vi "Keithley 6517 Perform Zero Correction_Cut.vi"(2 "Error In":errorcluster, 3 "VISA resource name":refnum<visa-resource-name>) -> (0 "Error Out":errorcluster, 1 "Measurement":T1 {"Measurement" format="%.6e"})   [LabVIEW 2016]
doc: "This example shows how to perform zero correction.\n\n<B>Note:</B>\nThis Example is compatible with both model 6517 and 6514."
uses:
  <instrlib>/Keithley 6517/Keithley 6517.lvlib
panel:
  in  "Instrument Model":i32(ring)=2 items=["MODEL 6517B", "MODEL 6517A", "MODEL 6514"]
  # "(c) 2016-2017 National Instruments.  ALL RIGHTS RESERVED."
  # "Note: This Example is compatible with model 6517 and 6514."
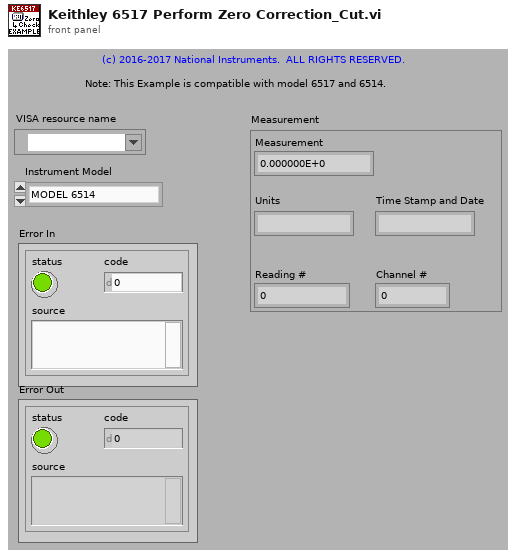
[diagram p1: front panel]
types:
  T1 = cluster{"Measurement":dbl, "Units":string, "Time Stamp and Date":string, "Reading #":dbl, "Channel #":dbl}
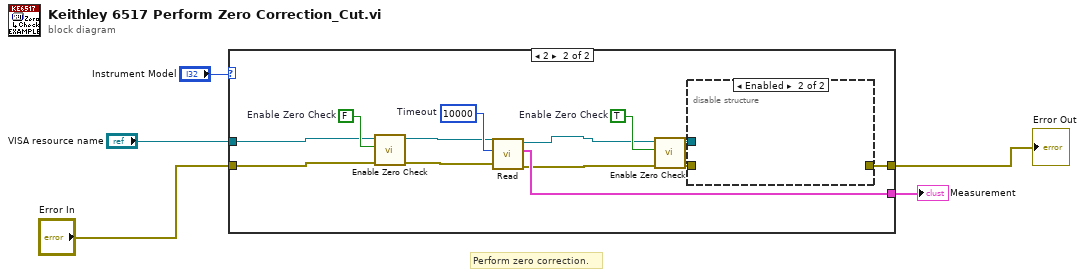
[diagram p0: block diagram]
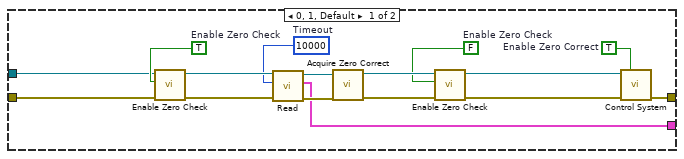
[diagram p2: hidden frame]
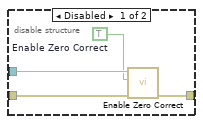
[diagram p3: hidden frame]
diagram:
  # "Perform zero correction."
  n1 = case shown="2" "Instrument Model" {
    tunnel: "VISA resource name" -> [w14 w32]
    tunnel: "Error In" -> [w13 w31]
    tunnel: [w12 w27] -> w1
    tunnel: [w6 w29] -> w5
    frame 0, 1, Default {
      w7 = u32 10000  # Timeout
      w17 = FALSE  # Enable Zero Check
      w20 = TRUE  # Enable Zero Correct
      w21 = TRUE  # Enable Zero Check
      n2 = call <instrlib>:"Enable Zero Check.vi"("error in (no error)"=w13, "Enable Zero Check (T: Enable)"=w21, "VISA resource name"=w14) -> ("error out"=w8:errorcluster, "VISA resource name out"=w9:refnum<visa-resource-name>)  [unwired: 7 in]
      n3 = call <instrlib>:"Read.vi"("error in (no error)"=w8, "Timeout(10000 ms)"=w7, "VISA resource name"=w9) -> ("error out"=w11:errorcluster, "Measurement"=w6:T1, "VISA resource name out"=w10:refnum<visa-resource-name>)  [unwired: 6 in]
      n4 = call <instrlib>:"Acquire Zero Correct.vi"("error in (no error)"=w11, "VISA resource name"=w10) -> ("error out"=w18:errorcluster, "VISA resource name out"=w19:refnum<visa-resource-name>)  [unwired: 8 in]
      n5 = call <instrlib>:"Enable Zero Check.vi"("error in (no error)"=w18, "Enable Zero Check (T: Enable)"=w17, "VISA resource name"=w19) -> ("error out"=w15:errorcluster, "VISA resource name out"=w16:refnum<visa-resource-name>)  [unwired: 7 in]
      n6 = call <instrlib>:"Control System.vi"("VISA resource name"=w16, "Enable Zero Correct (F: Disable)"=w20, "error in (no error)"=w15) -> ("error out"=w12:errorcluster)  [unwired: 11 in, 1 out]
    }
    frame 2 {
      w30 = u32 10000  # Timeout
      w33 = TRUE  # Enable Zero Check
      w34 = FALSE  # Enable Zero Check
      n7 = call <instrlib>:"Enable Zero Check.vi"("error in (no error)"=w31, "Enable Zero Check (T: Enable)"=w34, "VISA resource name"=w32) -> ("error out"=w22:errorcluster, "VISA resource name out"=w23:refnum<visa-resource-name>)  [unwired: 7 in]
      n8 = call <instrlib>:"Read.vi"("error in (no error)"=w22, "Timeout(10000 ms)"=w30, "VISA resource name"=w23) -> ("error out"=w24:errorcluster, "Measurement"=w29:T1, "VISA resource name out"=w25:refnum<visa-resource-name>)  [unwired: 6 in]
      n9 = call <instrlib>:"Enable Zero Check.vi"("error in (no error)"=w24, "Enable Zero Check (T: Enable)"=w33, "VISA resource name"=w25) -> ("error out"=w28:errorcluster, "VISA resource name out"=w26:refnum<visa-resource-name>)  [unwired: 7 in]
      n10 = disable-structure shown="Enabled" {
        disable-tunnel: w28 -> [w38 _]
        disable-tunnel: [w37 _] -> w27
        disable-tunnel: w26 -> [w36 _]
        frame Disabled {
          w35 = TRUE  # Enable Zero Correct
          n11 = call <instrlib>:"Enable Zero Correct.vi"("error in (no error)"=w38, "Enable Zero Correct (F: Disable)"=w35, "VISA resource name"=w36) -> ("error out"=w37:errorcluster)  [unwired: 7 in, 1 out]
        }
        frame Enabled {
        }
      }
    }
  }
  "Measurement" <- w5
  "Error Out" <- w1
